vi "Init.vi"(8 "error in (no error)":errorcluster, 10 "Instrument Ref":variant, 11 "APS 7050":refnum<class "APS 7050.lvclass">) -> (0 "error out":errorcluster, 2 "Found?":bool, 3 "APS 7050 out":refnum<class "APS 7050.lvclass">)   [LabVIEW 2025, in "Power Supply.lvlib" / "APS 7050.lvclass"]
uses:
  APS 7050.lvclass
  APS 7050.lvclass/APS 7050.ctl
  Users/Public/Documents/Sandia National Labs/TSS Plugin/Abstract Engine.lvlibp/Instrument configuration/Instrument configuration.lvclass
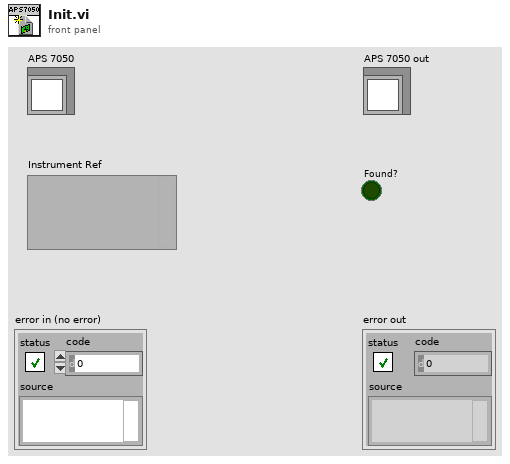
[diagram p1: front panel]
types:
  T1 = typedef "Abstract Engine.lvlibp/Instrument configuration.lvclass/Default Instrument.ctl" = cluster{"Type":string, "Address":string, "SW Alias":string, "Description":string, "Enabled":bool}
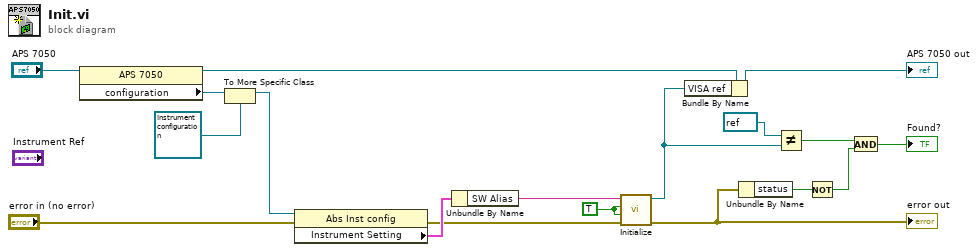
[diagram p0: block diagram]
diagram:
  w18 = TRUE ("ID Query (True)")
  n1 = property class="APS 7050"(reference="APS 7050") -> (reference out=w9:refnum<class "APS 7050.lvclass">, "configuration"=w14:refnum<class "CEF_serializable configuration.lvclass">)  [unwired: 1 in, 1 out]
  n2 = To More Specific Class(target class=refnum<class "Instrument configuration.lvclass"> refnum ("Abstract PlugIn.lvlibp:Instrument configuration"), reference=w14) -> (specific class reference=w13:refnum<class "Instrument configuration.lvclass">)  [unwired: 1 in, 1 out]
  n3 = property class="Abs Inst config"(reference=w13, error in="error in (no error)") -> (error out=w11:errorcluster, "Instrument Setting"=w16:T1)  [unwired: 1 out]
  n4 = Unbundle By Name(w16) -> ("SW Alias"=w8:string)
  n5 = call <instrlib>:"Initialize.vi"("error in (no error)"=w11, "Reset (True)"=w18, "ID Query (True)"=w18, "VISA resource name"=w8) -> ("error out"=w4:errorcluster, "VISA resource name out"=w3:refnum<visa-resource-name>)  [unwired: 6 in]
  "error out" <- w4
  n6 = Bundle By Name(cluster=w9, "VISA ref"=w3) -> (→"APS 7050 out":refnum<class "APS 7050.lvclass">)
  n7 = Unbundle By Name(w4) -> ("status"=w5:bool)
  n8 = Not Equal?(x=refnum<visa-resource-name> refnum ("VISA resource name out"), y=w3) -> (x != y?=w6:bool)
  n9 = Not(x=w5) -> (.not. x?=w7:bool)
  n10 = And(x=w6, y=w7) -> (x .and. y?=→"Found?":bool)
